vi "WriteConfigurationFile.vi"(8 "Error in":errorcluster, 10 "App Configuration":T1, 11 "Configuration File Path":path) -> (0 "Error out":errorcluster)   [LabVIEW 2019]
uses:
  #cluster_AppConfiguration.ctl
  <vilib>/Utility/config.llb/Write Key (Path).vi
  <vilib>/Utility/config.llb/NI_LVConfig.lvlib
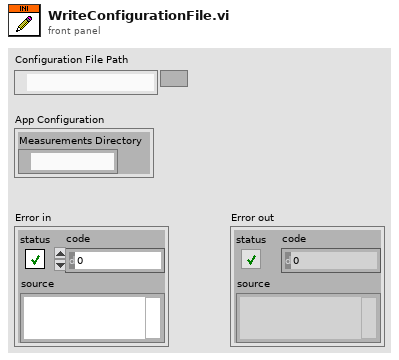
[diagram p1: front panel]
types:
  T1 = typedef "#cluster_AppConfiguration.ctl" = cluster{"Measurements Directory":path}
  T2 = typedef "NI_LVConfig.lvlib/Config Data RefNum.ctl" = refnum<k1>
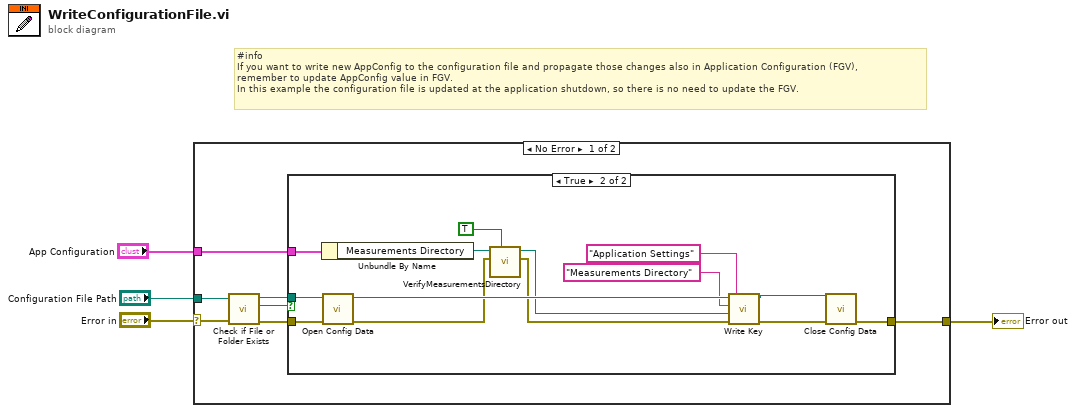
[diagram p0: block diagram]
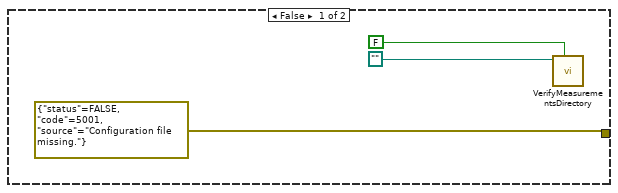
[diagram p2: hidden frame]
diagram:
  # "#info\nIf you want to write new AppConfig to the configuration file and propagate those changes also in Application Configuration (FGV),\nremember to update AppConfig value in FGV.\nIn this example the configuration file is updated at the application shutdown, so there is no need to update the FGV."
  n1 = case shown="No Error" "Error in" {
    selector: "Error in" -> [w7 w29]
    tunnel: "Configuration File Path" -> [w11 _]
    tunnel: [w6 w29] -> w2
    tunnel: "App Configuration" -> [w5 _]
    frame No Error {
      n2 = call <vilib>:"Check if File or Folder Exists.vi"("error in (no error)"=w7, "path"=w11) -> ("error out"=w9:errorcluster, "file or folder exists?"=w10:bool, "dup path"=w8:path)  [unwired: 7 in]
      n3 = case shown="True" w10 {
        tunnel: w9 -> [_ w27]
        tunnel: w8 -> [_ w28]
        tunnel: [errorcluster {"status"=FALSE, "code"=5001, "source"="Configuration file missing."} ("error constant") w23] -> w6
        tunnel: w5 -> [_ w20]
        frame False {
          n4 = call "VerifyMeasurementsDirectory.vi"("Key Found?"=FALSE, "Measurements Directory Path in"=path "") -> ()  [unwired: 8 in, 2 out]
        }
        frame True {
          n5 = Unbundle By Name(w20) -> ("Measurements Directory"=w19:path)
          n6 = call <vilib>:"Open Config Data.vi"("error in (no error)"=w27, "configuration file path"=w28) -> ("error out"=w17:errorcluster, "refnum"=w26:T2)  [unwired: 7 in, 1 out]
          n7 = call "VerifyMeasurementsDirectory.vi"("Key Found?"=TRUE, "Error in"=w17, "Measurements Directory Path in"=w19) -> ("Error out"=w16:errorcluster, "Measurements Directory Path out"=w15:path)  [unwired: 7 in]
          n8 = call-poly <vilib>:"Write Key.vi"("section"="Application Settings", "error in (no error)"=w16, "value"=w15, "key"="Measurements Directory" ("section"), "refnum"=w26) -> ("error out"=w22:errorcluster, "refnum out"=w21:T2)  [unwired: 4 in, 1 out]
          n9 = call <vilib>:"Close Config Data.vi"("error in (no error)"=w22, "refnum"=w21) -> ("error out"=w23:errorcluster)  [unwired: 8 in, 1 out]
        }
      }
    }
    frame Error {
    }
  }
  "Error out" <- w2
